vi "RIOchannelStorage.vi"(8 "Error in":errorcluster, 10 "Channel Settings":T1[][](array[typedef]), 11 "Tree DVR in":refnum<data-value>) -> (0 "Error out":errorcluster)   [LabVIEW 2014]
uses:
  Controls/RIOSettingsChannelSettings.ctl
  <vilib>/MDSplus/Classes/Tree_Class/Tree.lvclass
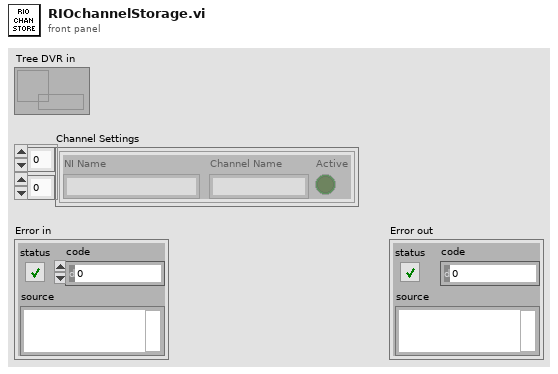
[diagram p1: front panel]
types:
  T1 = typedef "RIOSettingsChannelSettings.ctl" = cluster{"Channel Name":string, "Active":bool, "NI Name":string}
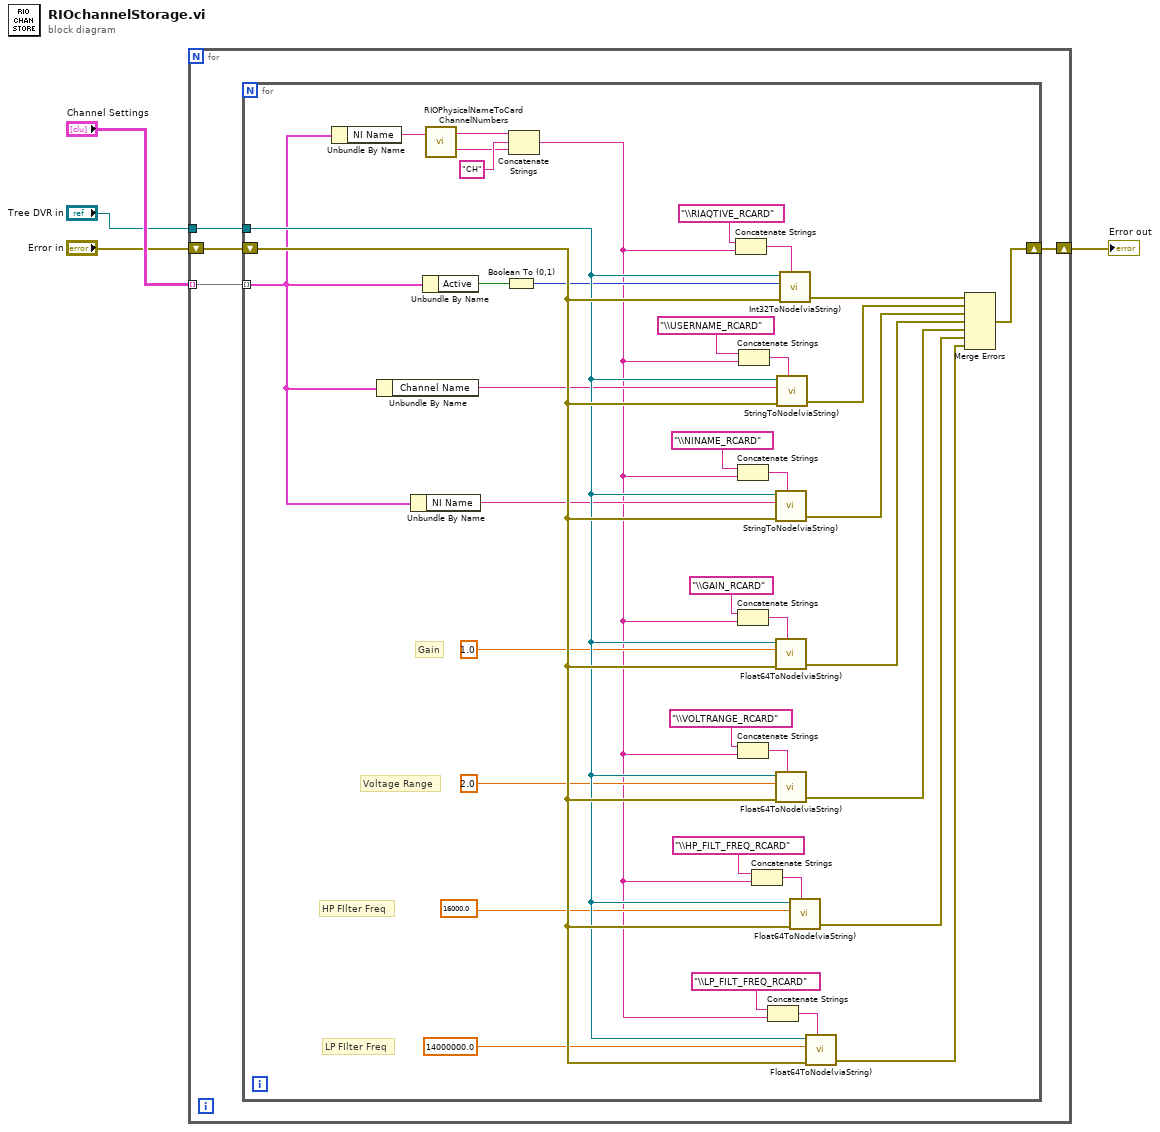
[diagram p0: block diagram]
diagram:
  n1 = for {
    tunnel: "Channel Settings" -> [w8] mode=indexing
    shift-right: [w7] -> w2
    shift-left: "Error in" -> [w5]
    tunnel: "Tree DVR in" -> [w6]
    n2 = for {
      tunnel: w8 -> [w43] mode=indexing
      tunnel: w6 -> [w44]
      shift-right: [w46] -> w7
      shift-left: w5 -> [w45]
      # "LP FIlter Freq"
      # "Voltage Range"
      # "HP FIlter Freq"
      # "Gain"
      n3 = Unbundle By Name(w43) -> ("NI Name"=w9:string)
      n4 = Unbundle By Name(w43) -> ("Channel Name"=w17:string)
      n5 = Unbundle By Name(w43) -> ("NI Name"=w16:string)
      n6 = Unbundle By Name(w43) -> ("Active"=w40:bool)
      n7 = call "RIOPhysicalNameToCardChannelNumbers.vi"("Channel Name"=w9) -> ("Channel #"=w11:string, "Card #"=w12:string)  [unwired: 1 in]
      n8 = Boolean To (0,1)(Boolean=w40) -> (0, 1=w39:i16)
      n9 = Concatenate Strings(w12, "CH" ("string"), w11) -> (w10:string)
      n10 = Concatenate Strings("\\RIAQTIVE_RCARD" ("string"), w10) -> (w37:string)
      n11 = Concatenate Strings("\\NINAME_RCARD" ("string"), w10) -> (w18:string)
      n12 = Concatenate Strings("\\GAIN_RCARD" ("string"), w10) -> (w25:string)
      n13 = Concatenate Strings("\\VOLTRANGE_RCARD" ("string"), w10) -> (w29:string)
      n14 = Concatenate Strings("\\USERNAME_RCARD" ("string"), w10) -> (w20:string)
      n15 = Concatenate Strings("\\HP_FILT_FREQ_RCARD" ("string"), w10) -> (w34:string)
      n16 = Concatenate Strings("\\LP_FILT_FREQ_RCARD" ("string"), w10) -> (w42:string)
      n17 = call "StringToNode(viaString).vi"("Tree DVR in"=w44, "String value in"=w16, "error in (no error)"=w45, "NodePath"=w18) -> ("error out"=w15:errorcluster)  [unwired: 2 in, 1 out]
      n18 = call "Float64ToNode(viaString).vi"("Tree DVR in"=w44, "DBL in"=1.0, "error in"=w45, "NodePath"=w25) -> ("error out"=w22:errorcluster)  [unwired: 2 in, 1 out]
      n19 = call "Float64ToNode(viaString).vi"("Tree DVR in"=w44, "DBL in"=2.0, "error in"=w45, "NodePath"=w29) -> ("error out"=w27:errorcluster)  [unwired: 2 in, 1 out]
      n20 = call "StringToNode(viaString).vi"("Tree DVR in"=w44, "String value in"=w17, "error in (no error)"=w45, "NodePath"=w20) -> ("error out"=w14:errorcluster)  [unwired: 2 in, 1 out]
      n21 = call "Int32ToNode(viaString).vi"("Tree DVR in"=w44, "I32 in"=w39, "error in (no error)"=w45, "NodePath"=w37) -> ("error out"=w36:errorcluster)  [unwired: 2 in, 1 out]
      n22 = call "Float64ToNode(viaString).vi"("Tree DVR in"=w44, "DBL in"=16000.0, "error in"=w45, "NodePath"=w34) -> ("error out"=w30:errorcluster)  [unwired: 2 in, 1 out]
      n23 = call "Float64ToNode(viaString).vi"("Tree DVR in"=w44, "DBL in"=14000000.0, "error in"=w45, "NodePath"=w42) -> ("error out"=w31:errorcluster)  [unwired: 2 in, 1 out]
      n24 = Merge Errors(w36, w14, w15, w22, w27, w30, w31) -> (w46:errorcluster)
    }
  }
  "Error out" <- w2
